vi "read_configuration.vi"(7 "force load?":bool=TRUE, 8 "error in (no error)":errorcluster, 10 "config cluster variant in (data type)":variant, 11 "path":path) -> (0 "error out":errorcluster, 2 "config cluster variant out (populated":variant)   [LabVIEW 2010]
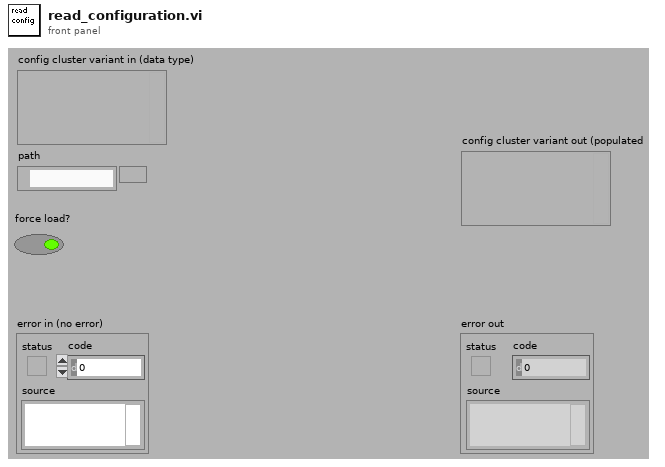
[diagram p1: front panel]
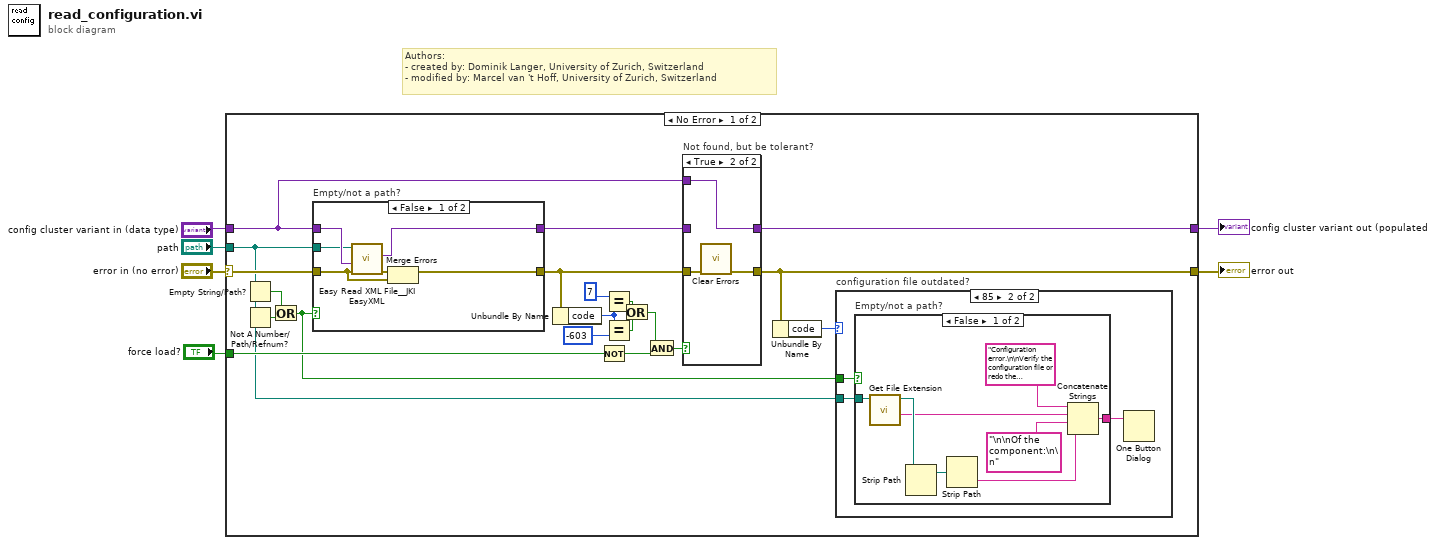
[diagram p0: block diagram]
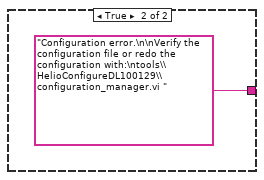
[diagram p3: hidden frame]
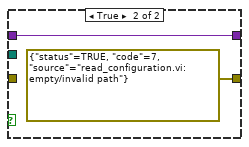
[diagram p4: hidden frame]
diagram:
  # "Authors: \n- created by: Dominik Langer, University of Zurich, Switzerland\n- modified by: Marcel van 't Hoff, University of Zurich, Switzerland"
  n1 = case shown="No Error" "error in (no error)" {
    selector: "error in (no error)" -> [w26 w52]
    tunnel: "config cluster variant in (data type)" -> [w12 w53]
    tunnel: "path" -> [w8 _]
    tunnel: [w9 w52] -> w3
    tunnel: [w10 w53] -> w2
    tunnel: "force load?" -> [w16 _]
    frame No Error {
      n2 = Empty String/Path?(string/path=w8) -> (empty?=w14:bool)
      n3 = Not A Number/Path/Refnum?(number/path/refnum=w8) -> (NaN/Path/Refnum?=w15:bool)
      n4 = Or(x=w14, y=w15) -> (x .or. y?=w7:bool)
      n5 = case "Empty/not a path?" shown="False" w7 {
        tunnel: w26 -> [w39 _]
        tunnel: w12 -> [w44 w46]
        tunnel: w8 -> [w43 _]
        tunnel: [w42 w46] -> w13
        tunnel: [w40 errorcluster {"status"=TRUE, "code"=7, "source"="read_configuration.vi: empty/invalid path"} ("error out")] -> w17
        frame False {
          n6 = call <vilib>:"Easy Read XML File__JKI EasyXML.vi"("error in (no error)"=w39, "LabVIEW Data (Type)"=w44, "XML File Path"=w43) -> ("error out"=w41:errorcluster, "LabVIEW Data"=w42:variant)  [unwired: 7 out]
          n7 = Merge Errors(w41, w39) -> (w40:errorcluster)
        }
        frame True {
        }
      }
      n8 = Unbundle By Name(w17) -> ("code"=w21:i32)
      n9 = Not(x=w16) -> (.not. x?=w19:bool)
      n10 = Equal?(x=7 ("y"), y=w21) -> (x = y?=w20:bool)
      n11 = Equal?(x=w21, y=-603) -> (x = y?=w24:bool)
      n12 = Or(x=w20, y=w24) -> (x .or. y?=w25:bool)
      n13 = And(x=w25, y=w19) -> (x .and. y?=w18:bool)
      n14 = case "Not found, but be tolerant?" shown="True" w18 {
        tunnel: w17 -> [w48 w51]
        tunnel: [w48 w50] -> w9
        tunnel: w13 -> [w47 _]
        tunnel: w12 -> [_ w49]
        tunnel: [w47 w49] -> w10
        frame False {
        }
        frame True {
          n15 = call <vilib>:"Clear Errors.vi"("error in (no error)"=w51) -> ("error out"=w50:errorcluster)  [unwired: 6 out]
        }
      }
      n16 = Unbundle By Name(w9) -> ("code"=w11:i32)
      n17 = case "configuration file outdated?" shown="85" w11 {
        tunnel: w8 -> [_ w28]
        tunnel: w7 -> [_ w27]
        frame Default {
        }
        frame 85 {
          n18 = case "Empty/not a path?" shown="False" w27 {
            tunnel: [w35 "Configuration error.\n\nVerify the configuration file or redo the configuration with:\ntools\\HelioConfigureDL100129\\configuration_manager.vi " ("message")] -> w29
            tunnel: w28 -> [w34 _]
            frame False {
              n19 = call <vilib>:"Get File Extension.vi"("file"=w34) -> ("filename without extension"=w32:string, "dup file"=w33:path)  [unwired: 7 in, 2 out]
              n20 = Strip Path(path=w33) -> (stripped path=w37:path)  [unwired: 1 out]
              n21 = Strip Path(path=w37) -> (name=w30:string)  [unwired: 1 out]
              n22 = Concatenate Strings("Configuration error.\n\nVerify the configuration file or redo the configuration with:\ntools\\HelioConfigureDL100129\\configuration_manager.vi \n\nMost likely it's caused by the configuration file:\n\n" ("message"), w32, "\n\nOf the component:\n\n" ("string"), w30) -> (w35:string)
            }
            frame True {
            }
          }
          n23 = One Button Dialog(message=w29) -> ()  [unwired: 1 in, 1 out]
        }
      }
    }
    frame Error {
    }
  }
  "config cluster variant out (populated" <- w2
  "error out" <- w3
